vi "Message Parameters FG.vi"(7 "Action":T3, 8 "error in (no error)":errorcluster, 10 "Message Settings":T1={"Generation Type"=enum."Trigger Only", "Period"=1.0, "Include Protection"=FALSE, "Type"=""}, 11 "Item Ref in":T4 format="%.0x") -> (0 "error out":errorcluster, 2 "Message Settings out":T1={"Generation Type"=enum."Trigger Only", "Period"=1.0, "Include Protection"=FALSE, "Type"=""}, 3 "Item Ref out":T4 format="%.0x")   [LabVIEW 2019, in "Instrument Addon Shared.lvlib"]
uses:
  Instrument Addon Shared.lvlib
  <vilib>/NI VeriStand/Custom Device API/Custom Device Item Ref.ctl
  Types/FG Control.ctl
  Types/Message Parameters.ctl
  Types/Message Generation Type.ctl
  Constants.vi
  <vilib>/NI VeriStand/Custom Device API/Get Item Property (U32).vi
  <vilib>/NI VeriStand/Custom Device API/Get Item Property (Double).vi
  <vilib>/NI VeriStand/Custom Device API/Get Item Property (Boolean).vi
  <vilib>/NI VeriStand/Custom Device API/Get Item Property (String).vi
  <vilib>/NI VeriStand/Custom Device API/Set Item Property (U32).vi
  <vilib>/NI VeriStand/Custom Device API/Set Item Property (Double).vi
  <vilib>/NI VeriStand/Custom Device API/Set Item Property (Boolean).vi
  <vilib>/NI VeriStand/Custom Device API/Set Item Property (String).vi
  <vilib>/NI VeriStand/Custom Device API/Custom Device API.lvlib
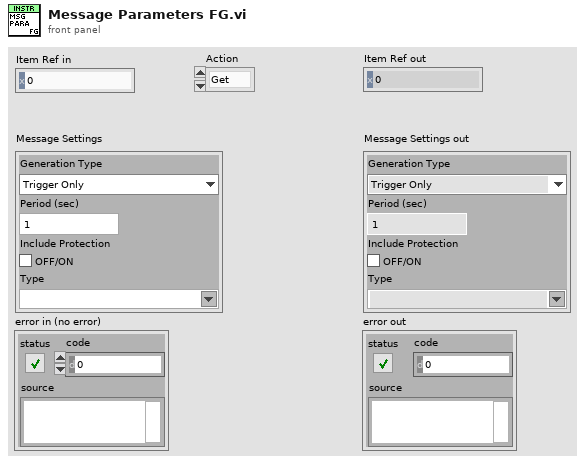
[diagram p1: front panel]
types:
  T1 = typedef "Instrument Addon Shared.lvlib/Message Parameters.ctl" = cluster{"Generation Type":T2, "Period":dbl, "Include Protection":bool, "Type":string}
  T2 = typedef "Instrument Addon Shared.lvlib/Message Generation Type.ctl" = enum16{"Trigger Only", "Periodic & Trigger", "Value Change & Trigger"}
  T3 = typedef "Instrument Addon Shared.lvlib/FG Control.ctl" = enum16{"Get", "Set"}
  T4 = typedef "Custom Device API.lvlib/Custom Device Item Ref.ctl" = u64
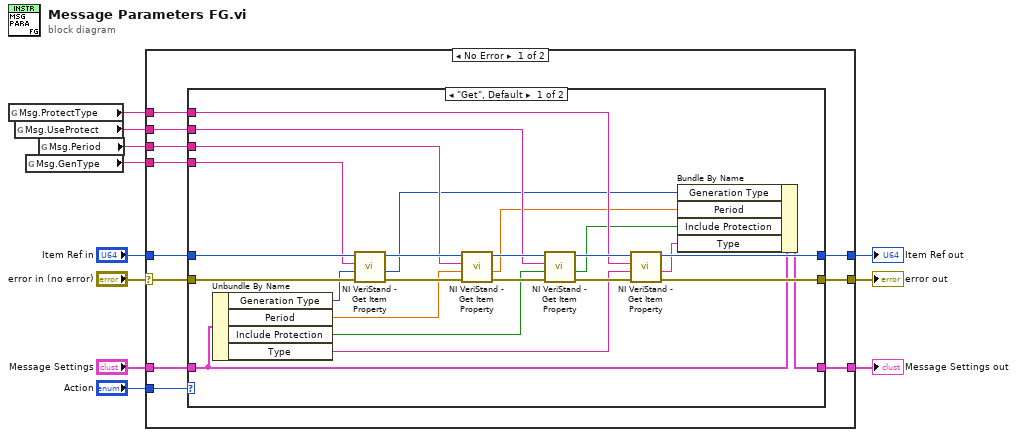
[diagram p0: block diagram]
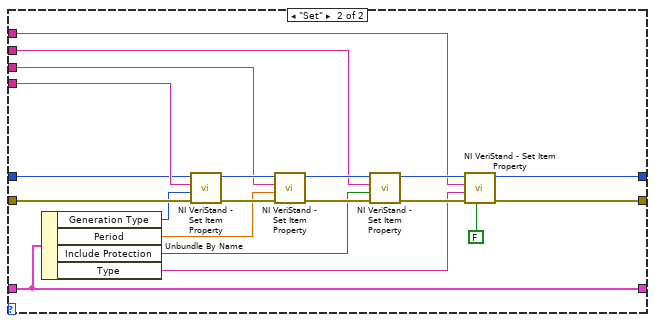
[diagram p2: hidden frame]
diagram:
  n1 = global read "Constants.vi" "Msg.ProtectType"() -> (w1:string)
  n2 = global read "Constants.vi" "Msg.UseProtect"() -> (w2:string)
  n3 = global read "Constants.vi" "Msg.GenType"() -> (w6:string)
  n4 = global read "Constants.vi" "Msg.Period"() -> (w3:string)
  n5 = case shown="No Error" "error in (no error)" {
    selector: "error in (no error)" -> [w17 w69]
    tunnel: w6 -> [w22 _]
    tunnel: [w21 w67] -> w9
    tunnel: "Item Ref in" -> [w20 w67]
    tunnel: "Message Settings" -> [w19 w68]
    tunnel: [w18 w69] -> w8
    tunnel: [w16 w68] -> w4
    tunnel: "Action" -> [w15 _]
    tunnel: w3 -> [w14 _]
    tunnel: w2 -> [w13 _]
    tunnel: w1 -> [w12 _]
    frame No Error {
      n6 = case shown="\"Get\", Default" w15 {
        tunnel: w22 -> [w44 w66]
        tunnel: [w39 w55] -> w21
        tunnel: w20 -> [w45 w65]
        tunnel: w19 -> [w24 w63]
        tunnel: [w40 w54] -> w18
        tunnel: w17 -> [w46 w64]
        tunnel: [w23 w63] -> w16
        tunnel: w14 -> [w31 w53]
        tunnel: w13 -> [w30 w52]
        tunnel: w12 -> [w29 w51]
        frame "Get", Default {
          n7 = Unbundle By Name(w24) -> ("Generation Type"=w35:T2, "Period"=w34:dbl, "Include Protection"=w33:bool, "Type"=w32:string)
          n8 = call-poly <vilib>:"NI VeriStand - Get Item Property.vi"("error in (no error)"=w46, "Default Value"=w35, "Property Name"=w44, "Item Ref in"=w45) -> ("error out"=w43:errorcluster, "Value"=w25:u32, "Item Ref out"=w36:T4)  [unwired: 4 in, 1 out]
          n9 = call-poly <vilib>:"NI VeriStand - Get Item Property.vi"("error in (no error)"=w43, "Default Value"=w34, "Property Name"=w31, "Item Ref in"=w36) -> ("error out"=w42:errorcluster, "Value"=w26:dbl, "Item Ref out"=w37:T4)  [unwired: 4 in, 1 out]
          n10 = call-poly <vilib>:"NI VeriStand - Get Item Property.vi"("error in (no error)"=w42, "Default Value"=w33, "Property Name"=w30, "Item Ref in"=w37) -> ("error out"=w41:errorcluster, "Value"=w27:bool, "Item Ref out"=w38:T4)  [unwired: 4 in, 1 out]
          n11 = call-poly <vilib>:"NI VeriStand - Get Item Property.vi"("error in (no error)"=w41, "Default Value"=w32, "Property Name"=w29, "Item Ref in"=w38) -> ("error out"=w40:errorcluster, "Value"=w28:string, "Item Ref out"=w39:T4)  [unwired: 4 in, 1 out]
          n12 = Bundle By Name(cluster=w24, "Generation Type"=w25, "Period"=w26, "Include Protection"=w27, "Type"=w28) -> (w23:T1)
        }
        frame "Set" {
          n13 = Unbundle By Name(w63) -> ("Generation Type"=w62:T2, "Period"=w47:dbl, "Include Protection"=w48:bool, "Type"=w49:string)
          n14 = call-poly <vilib>:"NI VeriStand - Set Item Property.vi"("error in (no error)"=w64, "Value"=w62, "Property Name"=w66, "Item Ref in"=w65) -> ("error out"=w61:errorcluster, "Item Ref out"=w58:T4)  [unwired: 5 in, 1 out]
          n15 = call-poly <vilib>:"NI VeriStand - Set Item Property.vi"("error in (no error)"=w61, "Value"=w47, "Property Name"=w53, "Item Ref in"=w58) -> ("error out"=w60:errorcluster, "Item Ref out"=w57:T4)  [unwired: 5 in, 1 out]
          n16 = call-poly <vilib>:"NI VeriStand - Set Item Property.vi"("error in (no error)"=w60, "Value"=w48, "Property Name"=w52, "Item Ref in"=w57) -> ("error out"=w59:errorcluster, "Item Ref out"=w56:T4)  [unwired: 5 in, 1 out]
          n17 = call-poly <vilib>:"NI VeriStand - Set Item Property.vi"("Binary String (T)"=FALSE, "error in (no error)"=w59, "Value"=w49, "Property Name"=w51, "Item Ref in"=w56) -> ("error out"=w54:errorcluster, "Item Ref out"=w55:T4)  [unwired: 4 in, 1 out]
        }
      }
    }
    frame Error {
    }
  }
  "error out" <- w8
  "Item Ref out" <- w9
  "Message Settings out" <- w4
